vi "current wip.vi"(8 "error in":errorcluster, 10 "LED INI":T1 {"Settings"."Source V" format="%#_g V"; "Settings"."VLED 3" format="%#_g V"; "Settings"."VLED 2" format="%#_g V"; "Settings"."VLED 1" format="%#f V"; "Limits"."Wavelength" format="%#_g nm"; "Limits"."Tolerance" format="%#_g %"; "Limits"."Current 3" format="%#_g  mA"; "Limits"."Current 2" format="%#_g  mA"; "Limits"."Current 1" format="%#_g mA"; "Instruments"."Resistor 3" format="%#_g ohm"; "Instruments"."Resistor 2" format="%#_g ohm"; "Instruments"."Resistor 1" format="%#f ohm"}, 11 "Test Visualize In":refnum<vi>) -> (0 "error out":errorcluster, 2 "Pass Fail":bool, 3 "Test Visualize Out":refnum<vi>)   [LabVIEW 2018]
uses:
  INI/INI File Control.ctl
  Public Controls/LVS Testplan.ctl
  Public Controls/LVS Instruments.ctl
  Public Controls/LVS Limits.ctl
  Public Controls/LVS Settings.ctl
  <vilib>/Analysis/6fits.llb/Curve Fitting Criteria.ctl
  <vilib>/Analysis/6fits.llb/General Linear Fit Algorithm.ctl
  <userlib>/_OpenG.lib/numeric/numeric.llb/Random Number Within Range - DBL__ogtk.vi
  <vilib>/Analysis/polynomials.llb/1D Polynomial Evaluation (DBL).vi
  <vilib>/Analysis/NI_AALPro.lvlib
  LED Control Module.lvlib
  INI/LED INI File.lvlib
panel:
  out "Array 3":bool[](array[boolean])
  out "Test Visualize":cluster{dbl[], dbl[]}[](graph)=[{[0.0, 0.0, 0.0], [0.0, nan, nan]}, {[-0.05, 0.0], [0.0, 0.0]}, {[-0.05, 0.0], [0.0, 0.0]}] caption="LED Current Consumption"
  # "Data Input"
  # "Local data"
  # "Data Output"
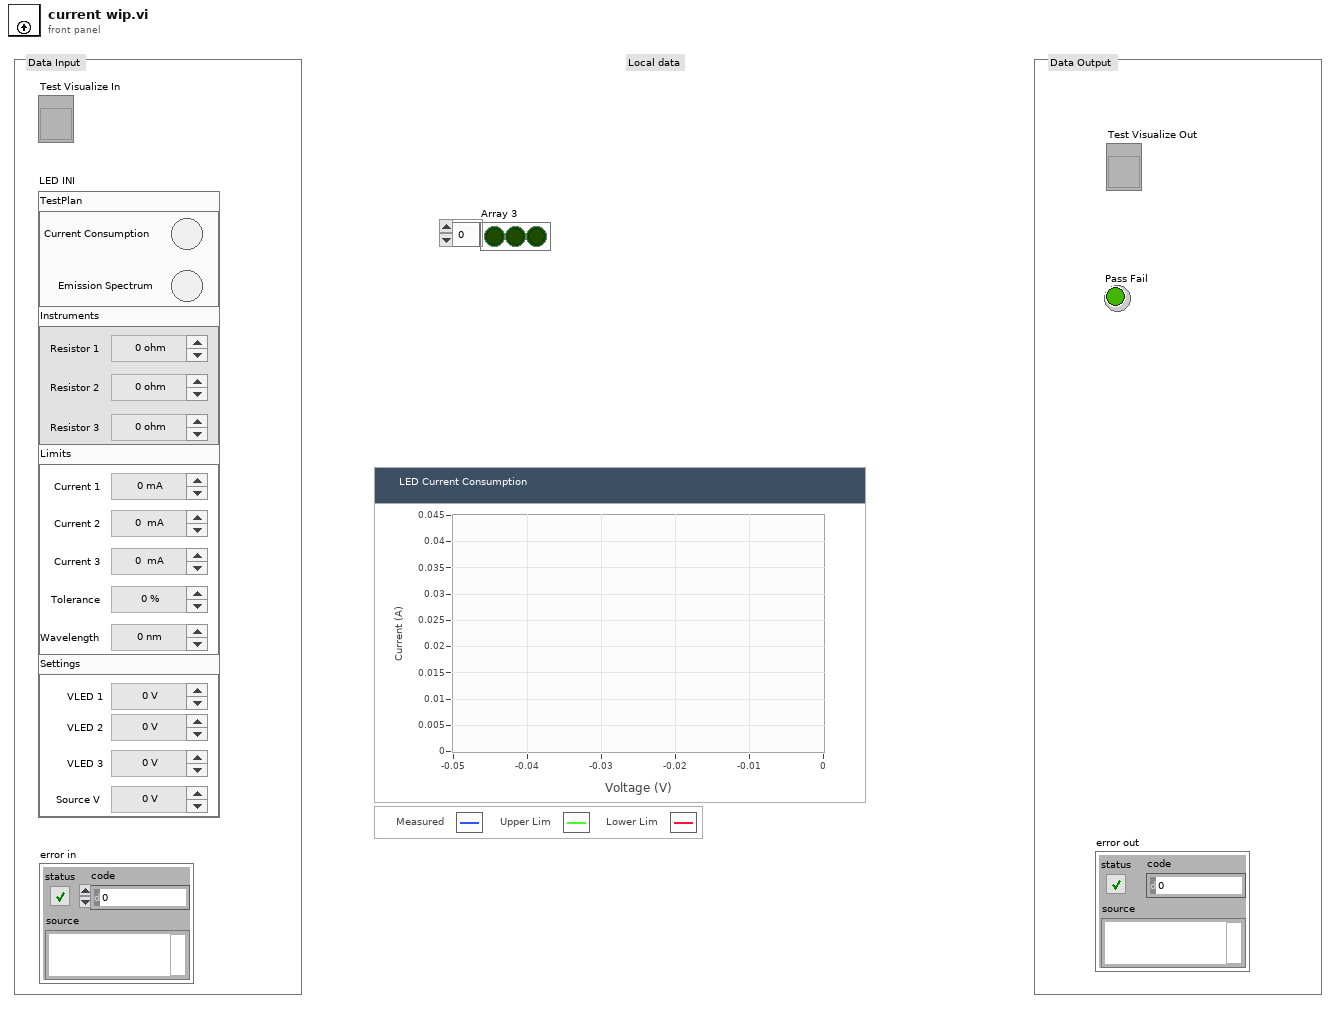
[diagram p1: front panel]
types:
  T1 = typedef "LED Control Module.lvlib/LED INI File.lvlib/INI File Control.ctl" = cluster{"TestPlan":T2, "Instruments":T3, "Limits":T4, "Settings":T5}
  T2 = typedef "LVS Testplan.ctl" = cluster{"Current Consumption":bool, "Emission Spectrum":bool}
  T3 = typedef "LED Control Module.lvlib/LVS Instruments.ctl" = cluster{"Resistor 1":dbl, "Resistor 2":dbl, "Resistor 3":dbl}
  T4 = typedef "LED Control Module.lvlib/LVS Limits.ctl" = cluster{"Current 1":dbl, "Current 2":dbl, "Current 3":dbl, "Tolerance":dbl, "Wavelength":dbl}
  T5 = typedef "LED Control Module.lvlib/LVS Settings.ctl" = cluster{"VLED 1":dbl, "VLED 2":dbl, "VLED 3":dbl, "Source V":dbl}
  T6 = cluster{"X Scale.Name Label.Text":string, "Y Scale.Name Label.Text":string, "Label.Text":string}
  T7 = typedef "NI_AALPro.lvlib/General Linear Fit Algorithm.ctl" = u16
  T8 = typedef "NI_AALPro.lvlib/Curve Fitting Criteria.ctl" = u16
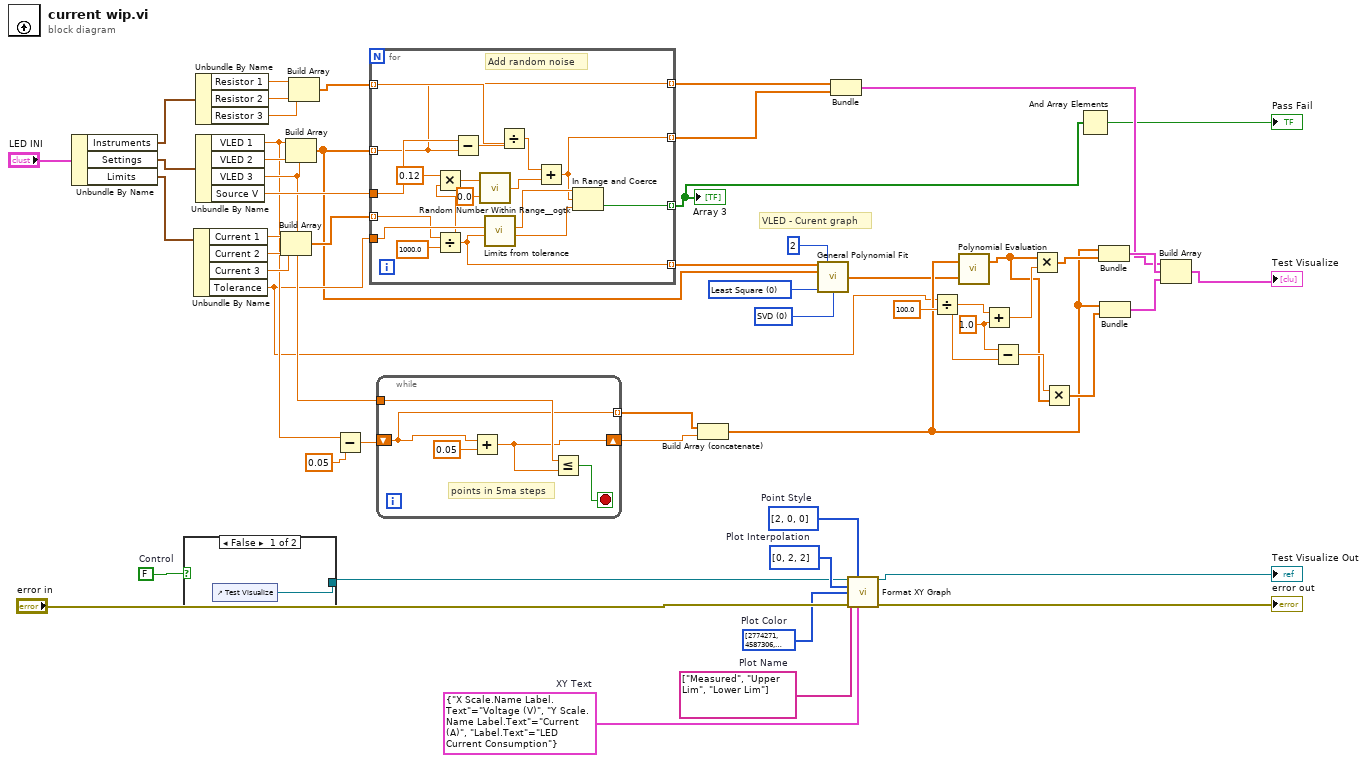
[diagram p0: block diagram]
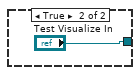
[diagram p2: hidden frame]
diagram:
  w14 = T6 {"X Scale.Name Label.Text"="Voltage (V)", "Y Scale.Name Label.Text"="Current (A)", "Label.Text"="LED Current Consumption"}  # XY Text
  w17 = FALSE  # Control
  w18 = string[] ["Measured", "Upper Lim", "Lower Lim"]  # Plot Name
  w19 = u32[] [2774271, 4587306, 16716354, 65351, 5898088, 3731200]  # Plot Color
  w20 = u8[] [0, 2, 2]  # Plot Interpolation
  w21 = u8[] [2, 0, 0]  # Point Style
  w43 = 1.0 ("y")
  w11 = T7 0 items=["SVD", "Givens", "Givens2", "Householder", "LU Decomposition", "Cholesky", "SVD for Rank Deficient H"] ("algorithm")
  w12 = T8 0 items=["Least Square", "Least Absolute Residual", "Bisquare"] ("method")
  # "VLED - Curent graph"
  n1 = Unbundle By Name("LED INI") -> ("Instruments"=w3:T3, "Settings"=w2:T5, "Limits"=w1:T4)
  n2 = case shown="False" w17 {
    tunnel: [w55 "Test Visualize In"] -> w16
    frame False {
      n3 = control-ref of="Test Visualize"() -> (w55:refnum<vi>)
    }
    frame True {
    }
  }
  n4 = Unbundle By Name(w1) -> ("Current 1"=w50:dbl, "Current 2"=w49:dbl, "Current 3"=w48:dbl, "Tolerance"=w15:dbl)
  n5 = Unbundle By Name(w3) -> ("Resistor 1"=w54:dbl, "Resistor 2"=w53:dbl, "Resistor 3"=w52:dbl)
  n6 = Unbundle By Name(w2) -> ("VLED 1"=w29:dbl, "VLED 2"=w51:dbl, "VLED 3"=w45:dbl, "Source V"=w46:dbl)
  n7 = Build Array(w50, w49, w48) -> (w13:dbl[])
  n8 = Build Array(w29, w51, w45) -> (w9:dbl[])
  n9 = Build Array(w54, w53, w52) -> (w47:dbl[])
  n10 = Subtract(x=w29, y=0.05) -> (x-y=w31:dbl)
  n11 = for {
    tunnel: w47 -> [w72] mode=indexing
    tunnel: w9 -> [w70] mode=indexing
    tunnel: w13 -> [w63] mode=indexing
    tunnel: w46 -> [w73]
    tunnel: [w58] -> w33 mode=indexing
    tunnel: [w70] -> w34 mode=indexing
    tunnel: w15 -> [w69]
    tunnel: [w67] -> w6 mode=indexing
    tunnel: [w57] -> w8 mode=indexing
    # "Add random noise"
    n12 = Divide(x=w63, y=1000.0) -> (x/y=w57:dbl)
    n13 = Multiply(x=0.12, y=w57) -> (x*y=w65:dbl)
    n14 = Subtract(x=w73, y=w70) -> (x-y=w71:dbl)
    n15 = call-poly <userlib>:"Random Number Within Range__ogtk.vi"("High"=w65, "Low"=0.0) -> ("Random Number"=w59:dbl)  [unwired: 3 in]
    n16 = call "Limits from tolerance.vi"("Nominal"=w57, "Tolerance %"=w69) -> ("Min Limit"=w61:dbl, "Max Limit"=w68:dbl)  [unwired: 8 in]
    n17 = Divide(x=w71, y=w72) -> (x/y=w60:dbl)
    n18 = Add(x=w60, y=w59) -> (x+y=w58:dbl)
    n19 = In Range and Coerce(upper limit=w68, x=w58, lower limit=w61) -> (In Range?=w67:bool)  [unwired: 1 out]
  }
  "Array 3" <- w6
  n20 = while {
    tunnel: w45 -> [w77]
    shift-right: [w76] -> w28
    shift-left: w31 -> [w74]
    tunnel: [w74] -> w27 mode=indexing
    stop <- w75 stop-if-true
    # "points in 5ma steps"
    n21 = Add(x=w74, y=0.05) -> (x+y=w76:dbl)
    n22 = Less Or Equal?(x=w77, y=w76) -> (x <= y?=w75:bool)
  }
  n23 = Build Array (concatenate)(w27, w28) -> (w26:dbl[])
  n24 = call <vilib>:"General Polynomial Fit.vi"("Y"=w8, "polynomial order"=2, "X"=w9, "method"=w12, "algorithm"=w11) -> ("Polynomial Coefficients"=w10:dbl[])  [unwired: 7 in, 3 out]
  n25 = Bundle(w34, w33) -> (w32:cluster{dbl[], dbl[]})  [unwired: 1 in]
  n26 = call "Format XY Graph.vi"("XYGraph in"=w16, "Point Style"=w21, "Plot Interpolation"=w20, "Plot Color"=w19, "Plot Name"=w18, "error in (no error)"="error in", "XY Text"=w14) -> ("XYGraph out"=→"Test Visualize Out":refnum<vi>, "error out"=→"error out":errorcluster)  [unwired: 7 in]
  n27 = Divide(x=w15, y=100.0) -> (x/y=w42:dbl)
  n28 = call-poly <vilib>:"Polynomial Evaluation.vi"("P(x)"=w10, "A"=w26) -> ("P(A)"=w39:dbl[])  [unwired: 1 out]
  n29 = Add(x=w42, y=w43) -> (x+y=w41:dbl)
  n30 = Subtract(x=w43, y=w42) -> (x-y=w40:dbl)
  n31 = Multiply(x=w39, y=w41) -> (x*y=w37:dbl[])
  n32 = Multiply(x=w40, y=w39) -> (x*y=w36:dbl[])
  n33 = And Array Elements(Boolean array=w6) -> (logical AND=→"Pass Fail":bool)
  n34 = Bundle(w26, w37) -> (w35:cluster{dbl[], dbl[]})  [unwired: 1 in]
  n35 = Bundle(w26, w36) -> (w38:cluster{dbl[], dbl[]})  [unwired: 1 in]
  n36 = Build Array(w32, w35, w38) -> (→"Test Visualize":cluster{dbl[], dbl[]}[])
